vi "1.3.3-Lidar Read Write.vi"   [LabVIEW 2010]
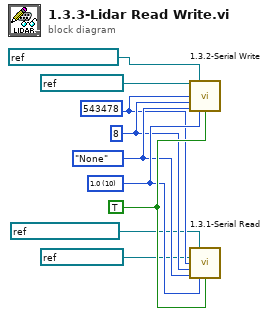
[diagram p0: block diagram]
diagram:
  w8 = TRUE ("Invert Polarity?")
  w7 = u16 10 items=["1.0"=10, "1.5"=15, "2.0"=20] ("stop bits (10: 1 bit)")
  w6 = enum16{"None", "Odd", "Even", "Mark", "Space"}."None" ("parity (0:none)")
  w5 = 8 ("data bits (8)")
  w4 = u32 543478 ("baud rate (9600)")
  n1 = call "1.3.2-Serial Write.vi"("Transmit"=refnum<k21> "Port4/DIO7", "Write FIFO"=refnum<k21> "2.3.1-Lidar Write", "baud rate (9600)"=w4, "data bits (8)"=w5, "parity (0:none)"=w6, "stop bits (10: 1 bit)"=w7, "Invert Polarity?"=w8) -> ()  [unwired: 9 in]
  n2 = call "1.3.1-Serial Read.vi"("Read FIFO"=refnum<k21> "2.3.2-Lidar Read", "Receive"=refnum<k21> "Port4/DIO8", "baud rate (9600)"=w4, "data bits (8)"=w5, "parity (0:none)"=w6, "stop bits (10: 1 bit)"=w7, "Invert Polarity?"=w8) -> ()  [unwired: 9 in]
